vi "test1-ListSubModulesInDifferentSenarios.vi"(8 "error in (no error)":errorcluster, 11 "TestCase in":refnum<class "testcase-CSMSubModule.lvclass">) -> (0 "error out":errorcluster, 3 "TestCase out":refnum<class "testcase-CSMSubModule.lvclass">)   [LabVIEW 2017, in "testcase-CSMSubModule.lvclass"]
uses:
  testcase-CSMSubModule.lvclass
  <vilib>/addons/_JKI Toolkits/VI Tester/TestCase.llb/TestCase.lvclass
  src/user.lib/_NEVSTOP/Communicable State Machine(CSM)/Communicable State Machine.lvlib
  C:/Program Files (x86)/National Instruments/LabVIEW 2017/vi.lib/addons/_JKI Toolkits/VI Tester/TestCase.llb/TestCase.lvclass
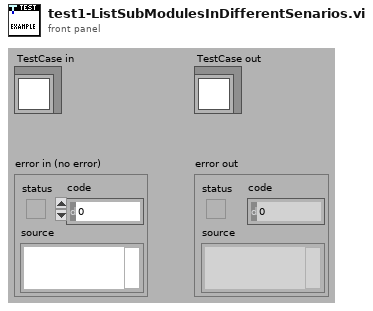
[diagram p1: front panel]
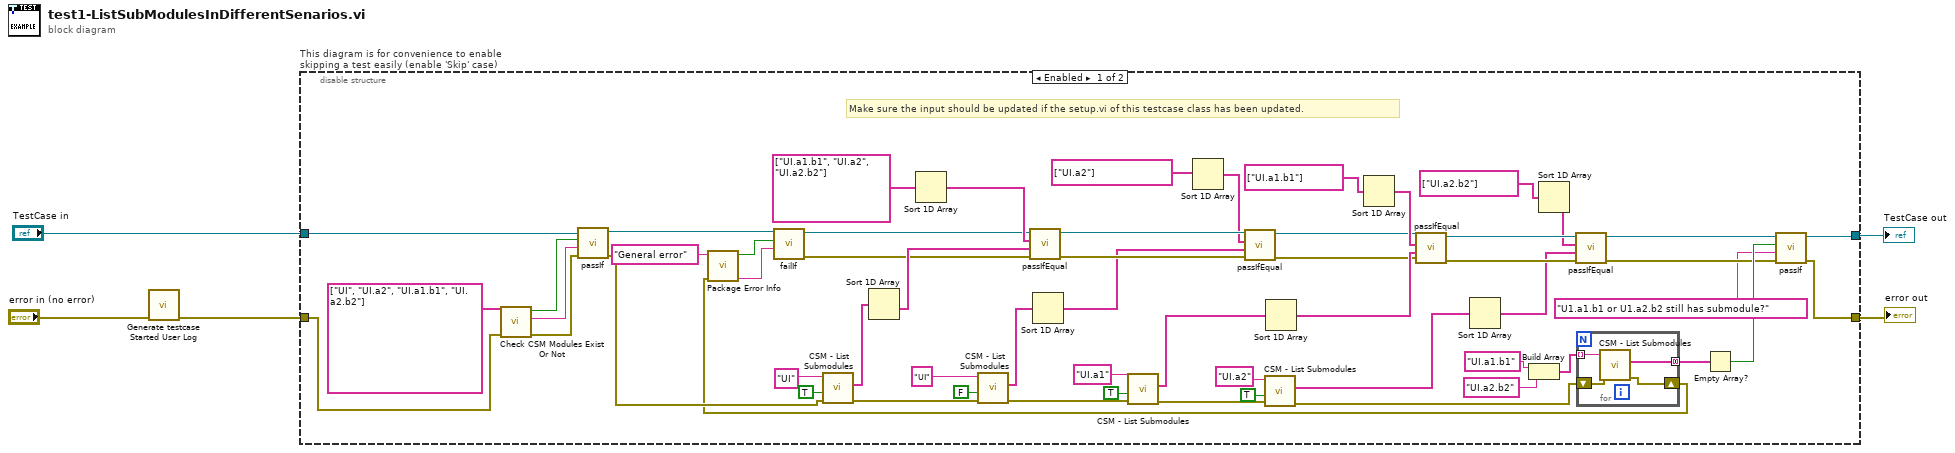
[diagram p0: block diagram]
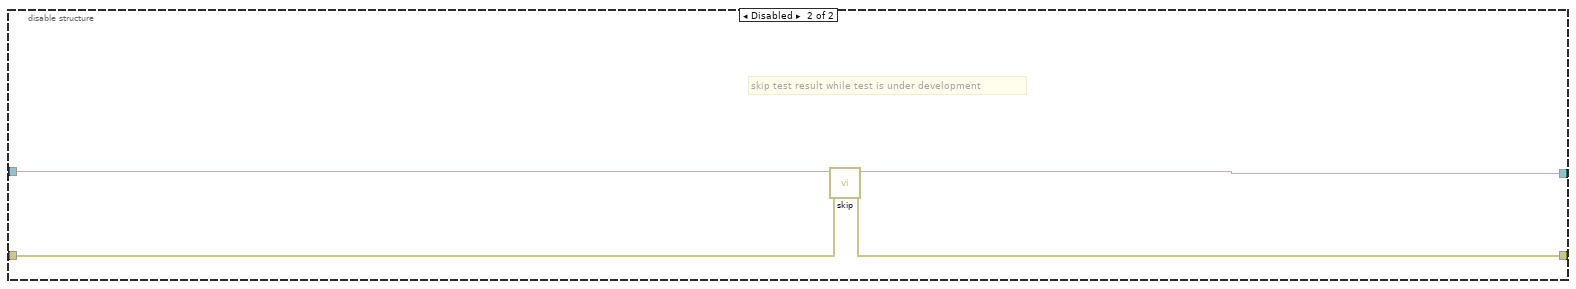
[diagram p2: hidden frame]
diagram:
  n1 = call "Generate testcase Started User Log.vi"("Error In"="error in (no error)") -> ("error out"=w1:errorcluster)  [unwired: 10 in]
  n2 = disable-structure "This diagram is for convenience to enable skipping a test easily (enable 'Skip' case)" shown="Enabled" {
    disable-tunnel: "TestCase in" -> [w16 w71]
    disable-tunnel: [w22 w69] -> w2
    disable-tunnel: [w21 w70] -> w4
    disable-tunnel: w1 -> [w15 w68]
    frame Enabled {
      # "Make sure the input should be updated if the setup.vi of this testcase class has been updated."
      n3 = call "Check CSM Modules Exist Or Not.vi"("error in"=w15, "CSM names in"=string[] ["UI", "UI.a2", "UI.a1.b1", "UI.a2.b2"]) -> ("error out"=w18:errorcluster, "Debug string"=w19:string, "All Modules Exist?"=w20:bool)  [unwired: 7 in]
      n4 = call-dynamic "passIf.vi"("error in (no error)"=w18, "message (\"\")"=w19, "pass"=w20, "TestCase in"=w16) -> ("error out"=w14:errorcluster, "TestCase out"=w11:refnum<class "testcase-CSMSubModule.lvclass">)  [unwired: 6 in]
      n5 = call "CSM - List Submodules.vi"("Error In"=w14, "Recursive? (T)"=TRUE, "Parent Name"="UI" ("Name (\"\" to Use UUID)")) -> ("Error Out"=w61:errorcluster, "Submodules"=w63:string[])  [unwired: 6 in, 1 out]
      n6 = Sort 1D Array(array=w63) -> (sorted array=w49:string[])
      n7 = Sort 1D Array(array=string[] ["UI.a1.b1", "UI.a2", "UI.a2.b2"] ("UI's Submodules 2")) -> (sorted array=w50:string[])
      n8 = call "CSM - List Submodules.vi"("Error In"=w61, "Recursive? (T)"=FALSE, "Parent Name"="UI" ("Name (\"\" to Use UUID)")) -> ("Error Out"=w59:errorcluster, "Submodules"=w48:string[])  [unwired: 6 in, 1 out]
      n9 = Sort 1D Array(array=w48) -> (sorted array=w45:string[])
      n10 = call "CSM - List Submodules.vi"("Error In"=w59, "Recursive? (T)"=TRUE, "Parent Name"="UI.a1" ("Name (\"\" to Use UUID)")) -> ("Error Out"=w57:errorcluster, "Submodules"=w40:string[])  [unwired: 6 in, 1 out]
      n11 = Sort 1D Array(array=string[] ["UI.a2"] ("UI's Submodules 2")) -> (sorted array=w43:string[])
      n12 = call "CSM - List Submodules.vi"("Error In"=w57, "Recursive? (T)"=TRUE, "Parent Name"="UI.a2" ("Name (\"\" to Use UUID)")) -> ("Error Out"=w27:errorcluster, "Submodules"=w34:string[])  [unwired: 6 in, 1 out]
      n13 = Sort 1D Array(array=w40) -> (sorted array=w39:string[])
      n14 = Sort 1D Array(array=string[] ["UI.a1.b1"] ("UI's Submodules 2")) -> (sorted array=w42:string[])
      n15 = Sort 1D Array(array=w34) -> (sorted array=w33:string[])
      n16 = Build Array("UI.a1.b1" ("Name (\"\" to Use UUID)"), "UI.a2.b2" ("Name (\"\" to Use UUID)")) -> (w28:string[])
      n17 = Sort 1D Array(array=string[] ["UI.a2.b2"] ("UI's Submodules 2")) -> (sorted array=w31:string[])
      n18 = for {
        tunnel: w28 -> [w67] mode=indexing
        shift-right: [w65] -> w8
        shift-left: w27 -> [w66]
        tunnel: [w64] -> w26 mode=concatenating
        n19 = call "CSM - List Submodules.vi"("Error In"=w66, "Parent Name"=w67) -> ("Error Out"=w65:errorcluster, "Submodules"=w64:string[])  [unwired: 7 in, 1 out]
      }
      n20 = call "Package Error Info.vi"("error in"=w8, "String in"="General error") -> ("packed error info out"=w12:string, "error status"=w13:bool)  [unwired: 8 in]
      n21 = call-dynamic "failIf.vi"("message (\"\")"=w12, "fail"=w13, "TestCase in"=w11) -> ("error out"=w9:errorcluster, "TestCase out"=w10:refnum<class "testcase-CSMSubModule.lvclass">)  [unwired: 7 in]
      n22 = call-dynamic "passIfEqual.vi"("error in (no error)"=w9, "y"=w49, "x"=w50, "TestCase in"=w10) -> ("error out"=w46:errorcluster, "TestCase out"=w47:refnum<class "testcase-CSMSubModule.lvclass">)  [unwired: 6 in]
      n23 = call-dynamic "passIfEqual.vi"("error in (no error)"=w46, "y"=w45, "x"=w43, "TestCase in"=w47) -> ("error out"=w37:errorcluster, "TestCase out"=w38:refnum<class "testcase-CSMSubModule.lvclass">)  [unwired: 6 in]
      n24 = call-dynamic "passIfEqual.vi"("error in (no error)"=w37, "y"=w39, "x"=w42, "TestCase in"=w38) -> ("error out"=w35:errorcluster, "TestCase out"=w36:refnum<class "testcase-CSMSubModule.lvclass">)  [unwired: 6 in]
      n25 = call-dynamic "passIfEqual.vi"("error in (no error)"=w35, "y"=w33, "x"=w31, "TestCase in"=w36) -> ("error out"=w23:errorcluster, "TestCase out"=w24:refnum<class "testcase-CSMSubModule.lvclass">)  [unwired: 6 in]
      n26 = Empty Array?(array=w26) -> (empty?=w25:bool)
      n27 = call-dynamic "passIf.vi"("error in (no error)"=w23, "message (\"\")"="U1.a1.b1 or U1.a2.b2 still has submodule?" ("message (\"\")"), "pass"=w25, "TestCase in"=w24) -> ("error out"=w21:errorcluster, "TestCase out"=w22:refnum<class "testcase-CSMSubModule.lvclass">)  [unwired: 6 in]
    }
    frame Disabled {
      # "skip test result while test is under development"
      n28 = call <vilib>:"skip.vi"("error in (no error)"=w68, "TestCase in"=w71) -> ("error out"=w70:errorcluster, "TestCase out"=w69:refnum<class "testcase-CSMSubModule.lvclass">)  [unwired: 8 in]
    }
  }
  "error out" <- w4
  "TestCase out" <- w2
